vi "SetMTPFolder.vi"(1 "MTP Files in":cluster{"Motor ID":i32, "Tuning File":path}[](array[cluster]), 2 "MTP Folder (C:\\MotorParam)":path=path "C:/MotorParam") -> (0 "MTP Files out":cluster{"Motor ID":i32, "Tuning File":path}[](array[cluster]))   [LabVIEW 2016]
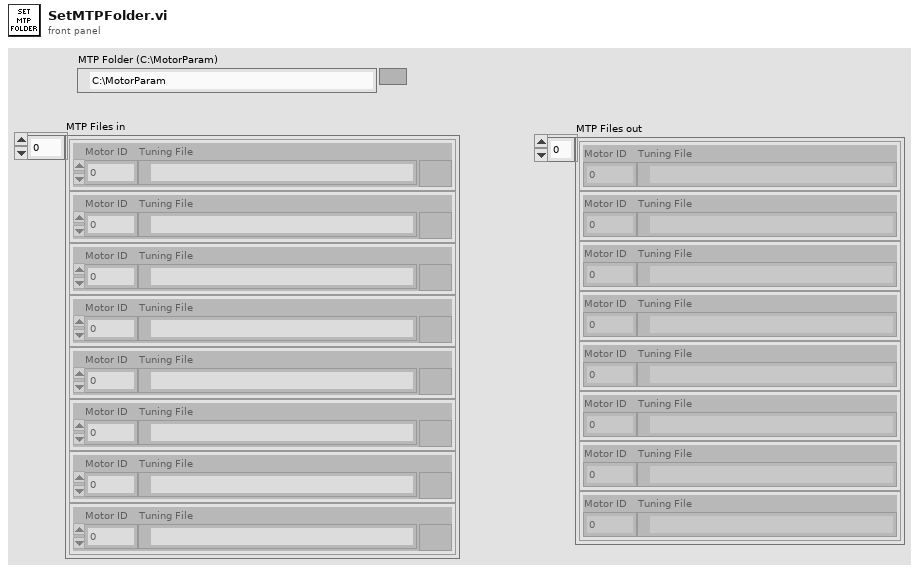
[diagram p1: front panel]
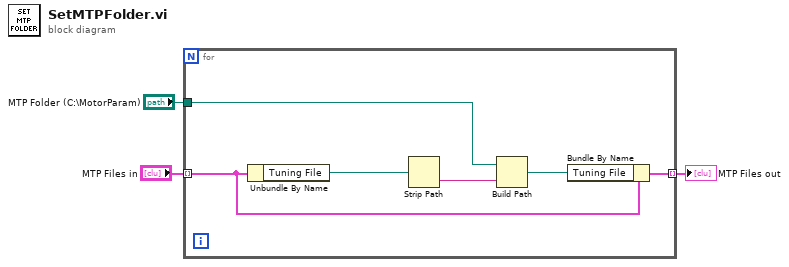
[diagram p0: block diagram]
diagram:
  n1 = for {
    tunnel: "MTP Files in" -> [w6] mode=indexing
    tunnel: "MTP Folder (C:\\MotorParam)" -> [w7]
    tunnel: [w4] -> w2 mode=indexing
    n2 = Unbundle By Name(w6) -> ("Tuning File"=w9:path)
    n3 = Strip Path(path=w9) -> (name=w8:string)  [unwired: 1 out]
    n4 = Build Path(base path=w7, name or relative path=w8) -> (appended path=w5:path)
    n5 = Bundle By Name(cluster=w6, "Tuning File"=w5) -> (w4:cluster{"Motor ID":i32, "Tuning File":path})
  }
  "MTP Files out" <- w2
